vi "2D U16 Array Changed__ogtk.vi"(1 "2D U16 Array":u16[][](array[numeric])) -> (0 "Changed":bool)   [LabVIEW 2017]
doc: "<B>Data Changed</B>\nThis is a polymorphic VI that will output a true if the data flowing into it has changed. It is also a Reentrant VI. So each intance of it in your code is treated as a seperate VI. The first time that the VI is run it will output a false. It can take any data type as an input. It has several native data types (for efficiency) and will coerce to variant if a non-native data type (error cluster, refnum, etc) is used."
panel:
  # "[OpenG VI Tags] ***Do Not Remove***"
  # "Data Changed.vi\n\nThis VI is used to detect whether the input has changed value.\n\nPlease visit http://www.OpenG.org to learn about the\nOpen Source LabVIEW software movement.\n\nNOTICE -- YOU MUST LEAVE THIS NOTICE IN PLACE.  PER THE TERMS OF THE LICENSE BELOW, YOU MAY SUBLICENSE THIS SOFTWARE \nIN ANY WAY THAT DOES NOT CONFLICT WITH THIS LICENSE.\n\n### BSD License (http://www.opensource.org/licenses/bsd-license.php) Begin ###\n \nCopyright (c) 2002, Jim Kring <jim@jimkring.com>\nCopyright (c) 2002, Cal-Bay Systems, Inc. <info@cal-bay.com>\n\nAll rights reserved.\n\nRedistribution and use in source and binary forms, with or without modification, are permitted provided that the following conditions are met:\n\n    * Redistributions of source code must retain the above copyright notice, this list of conditions and the following disclaimer.\n    * Redistributions in binary form must reproduce the above copyright notice, this list of conditions and the following disclaimer in the \n       documentation and/or other materials provided with the distribution.\n    * Neither the name of SciWare, James Kring, Inc., nor the names of its contributors may be used to endorse or promote products derived \n       from this software without specific prior written permission.\n\nTHIS SOFTWARE IS PROVIDED BY THE COPYRIGHT HOLDERS AND CONTRIBUTORS \"AS IS\" AND ANY EXPRESS OR IMPLIED WARRANTIES, \nINCLUDING, BUT NOT LIMITED TO, THE IMPLIED WARRANTIES OF MERCHANTABILITY AND FITNESS FOR A PARTICULAR PURPOSE ARE \nDISCLAIMED. IN NO EVENT SHALL THE COPYRIGHT OWNER OR CONTRIBUTORS BE LIABLE FOR ANY DIRECT, INDIRECT, INCIDENTAL,\n SPECIAL, EXEMPLARY, OR CONSEQUENTIAL DAMAGES (INCLUDING, BUT NOT LIMITED TO, PROCUREMENT OF SUBSTITUTE GOODS OR \nSERVICES; LOSS OF USE, DATA, OR PROFITS; OR BUSINESS INTERRUPTION) HOWEVER CAUSED AND ON ANY THEORY OF LIABILITY, \nWHETHER IN CONTRACT, STRICT LIABILITY, OR TORT (INCLUDING NEGLIGENCE OR OTHERWISE) ARISING IN ANY WAY OUT OF THE USE \nOF THIS SOFTWARE, EVEN IF ADVISED OF THE POSSIBILITY OF SUCH DAMAGE.\n\n### BSD License End ###"
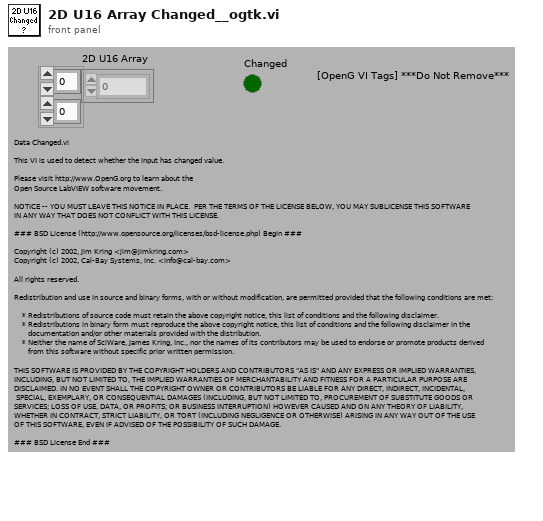
[diagram p1: front panel]
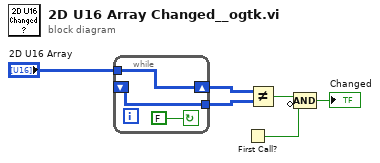
[diagram p0: block diagram]
diagram:
  n1 = while {
    shift-right: [w9] -> w6
    shift-left: _ -> [w8]
    tunnel: "2D U16 Array" -> [w9]
    tunnel: [w8] -> w5
    stop <- FALSE continue-if-true
  }
  n2 = First Call?() -> (First Call?: T/F=w1:bool)
  n3 = Not Equal?(x=w6, y=w5) -> (x != y?=w4:bool)
  n4 = Compound Arithmetic op=AND(w4, invert w1) -> (→"Changed":bool)
